vi "_UnitTest.GetDataTypeDescription.vi"() -> ()   [LabVIEW 2014]
panel:
  out "String 12":string
  out "String 16":string
  out "String 11":string
  out "String 15":string
  out "String 14":string
  in  "Digital Data":digitaldata
  out "String 13":string
  in  "Digital Waveform":digitalwaveform(waveform)={"t0"=timestamp(0 s since 1904-01-01), "dt"=1.0, "Y"={"transitions"=[], "data"=[]}}
  out "String 10":string
  in  "Enum":enum16{"a", "b", "c", "d"}(ring)
  out "String 9":string
  in  "Cluster 5":T1
  out "String 8":string
  in  "Cluster 4":T2
  out "String 7":string
  in  "Waveform":waveform(i32)
  out "String 5":string
  in  "Cluster 3":T3
  out "String 4":string
  in  "Cluster 2":T4
  out "String 3":string
  in  "Cluster":cluster{i32, dbl, enum16{""}}
  in  "Array":cluster{i32, dbl, enum16{""}}[](array[cluster])
  in  "Numeric":i32
  out "String 2":string
  out "String":string
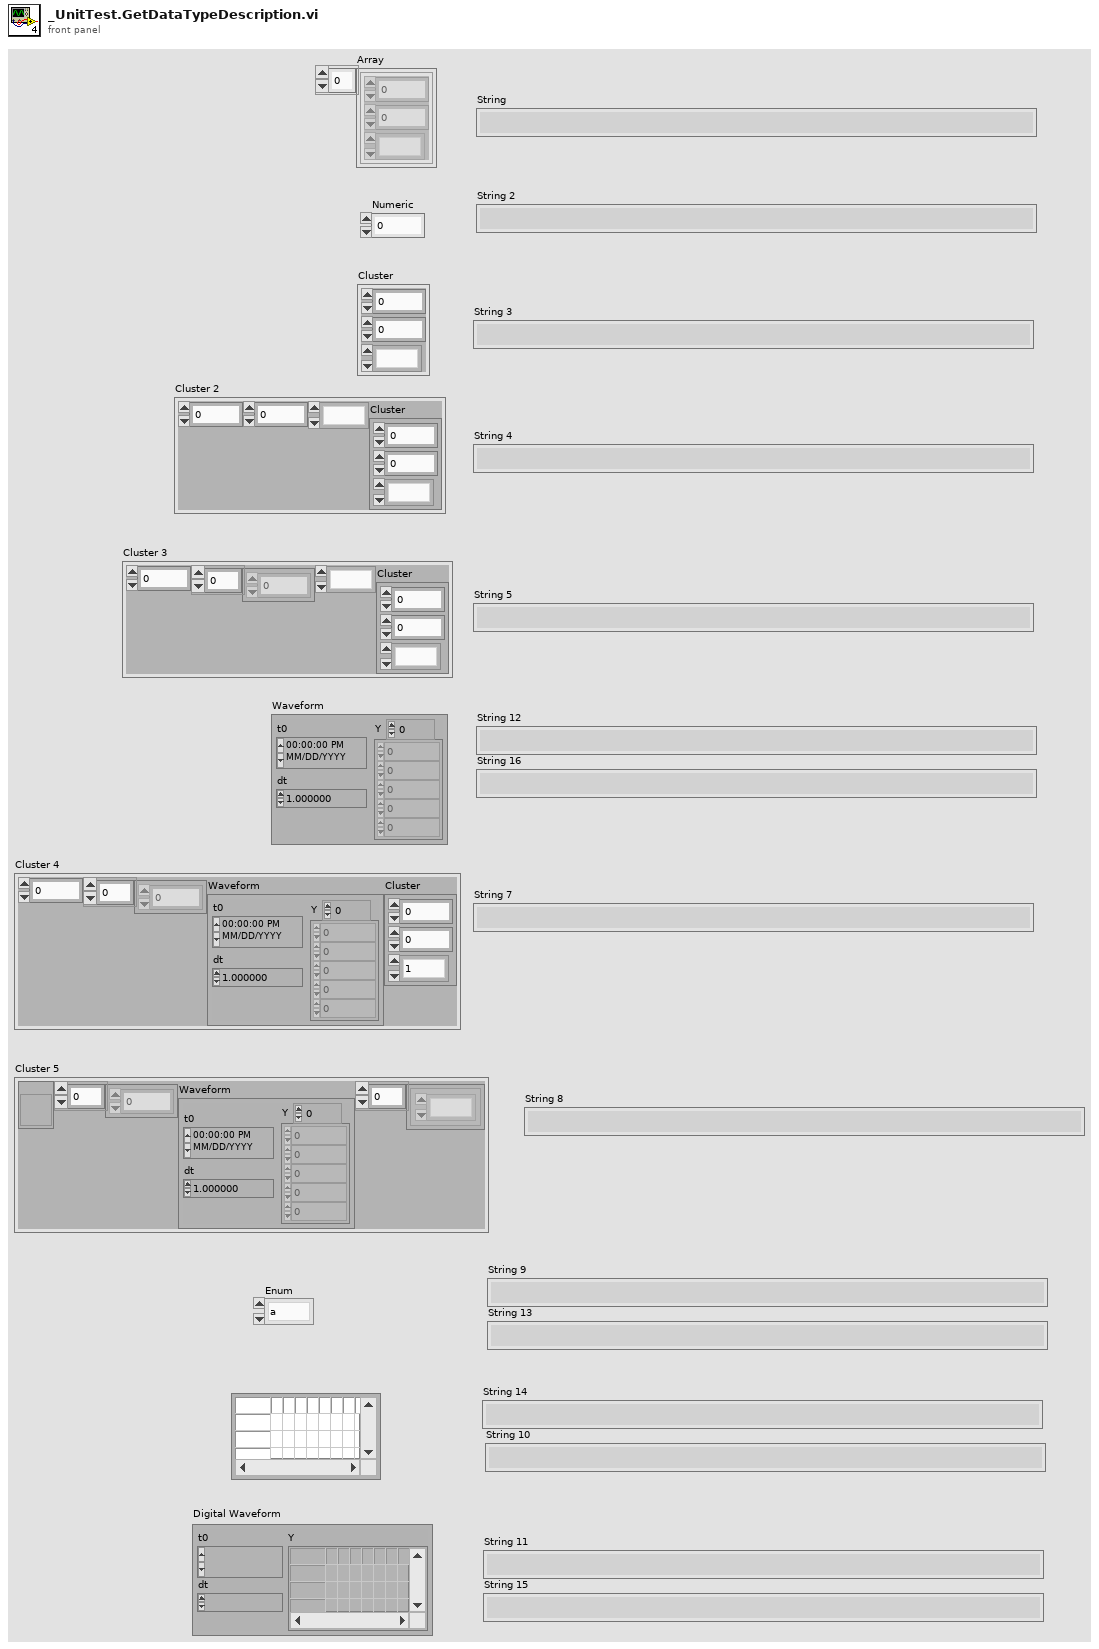
[diagram p1: front panel]
types:
  T1 = cluster{refnum<vi>, dbl[], "Waveform":waveform(dbl), refnum<k1>[]}
  T2 = cluster{i32, dbl[], "Waveform":waveform(dbl), "Cluster":cluster{i32, dbl, enum16{"1", "2", "3"}}}
  T3 = cluster{i32, dbl[], enum16{""}, "Cluster":cluster{i32, dbl, enum16{""}}}
  T4 = cluster{i32, dbl, enum16{""}, "Cluster":cluster{i32, dbl, enum16{""}}}
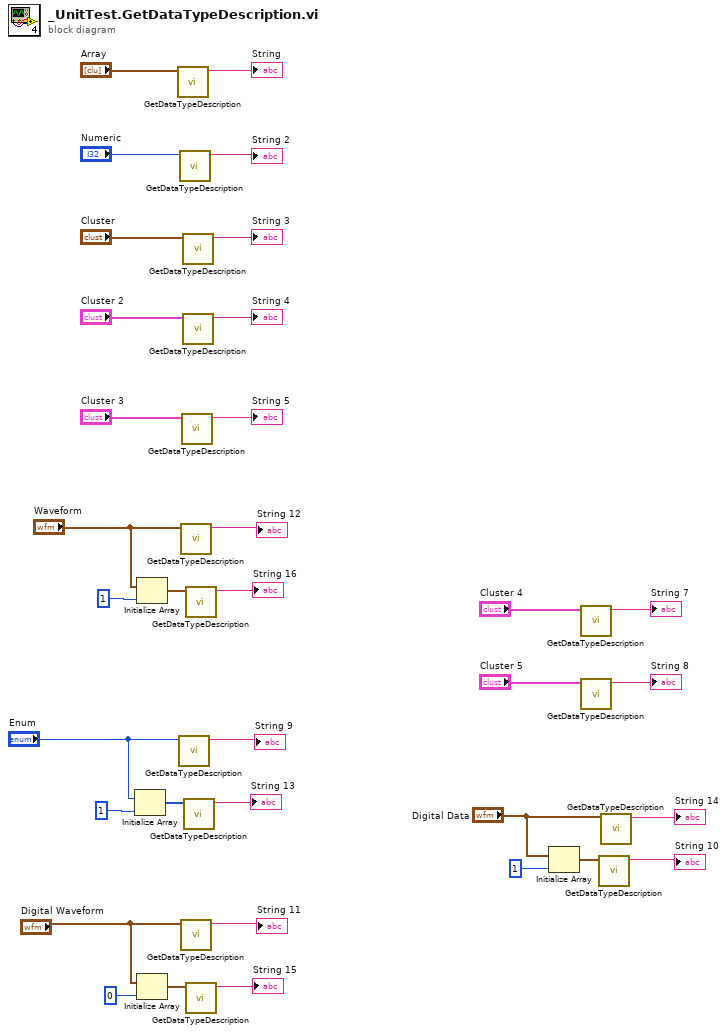
[diagram p0: block diagram]
diagram:
  n1 = Initialize Array("Enum", 1 ("dimension size")) -> (w11:enum16{"a", "b", "c", "d"}[])
  n2 = Initialize Array("Waveform", 1 ("dimension size")) -> (w5:waveform(i32)[])
  n3 = Initialize Array("Digital Waveform", 0 ("dimension size")) -> (w10:digitalwaveform[])
  n4 = call "GetDataTypeDescription.vi"("Variant"="Array") -> ("String"=→"String":string)  [unwired: 9 in, 1 out]
  n5 = call "GetDataTypeDescription.vi"("Variant"="Enum") -> ("String"=→"String 9":string)  [unwired: 9 in, 1 out]
  n6 = call "GetDataTypeDescription.vi"("Variant"="Numeric") -> ("String"=→"String 2":string)  [unwired: 9 in, 1 out]
  n7 = call "GetDataTypeDescription.vi"("Variant"="Waveform") -> ("String"=→"String 12":string)  [unwired: 9 in, 1 out]
  n8 = call "GetDataTypeDescription.vi"("Variant"="Digital Waveform") -> ("String"=→"String 11":string)  [unwired: 9 in, 1 out]
  n9 = call "GetDataTypeDescription.vi"("Variant"="Cluster 3") -> ("String"=→"String 5":string)  [unwired: 9 in, 1 out]
  n10 = call "GetDataTypeDescription.vi"("Variant"="Cluster") -> ("String"=→"String 3":string)  [unwired: 9 in, 1 out]
  n11 = call "GetDataTypeDescription.vi"("Variant"="Cluster 2") -> ("String"=→"String 4":string)  [unwired: 9 in, 1 out]
  n12 = call "GetDataTypeDescription.vi"("Variant"=w11) -> ("String"=→"String 13":string)  [unwired: 9 in, 1 out]
  n13 = call "GetDataTypeDescription.vi"("Variant"=w5) -> ("String"=→"String 16":string)  [unwired: 9 in, 1 out]
  n14 = call "GetDataTypeDescription.vi"("Variant"=w10) -> ("String"=→"String 15":string)  [unwired: 9 in, 1 out]
  n15 = Initialize Array("Digital Data", 1 ("dimension size")) -> (w15:digitaldata[])
  n16 = call "GetDataTypeDescription.vi"("Variant"="Cluster 4") -> ("String"=→"String 7":string)  [unwired: 9 in, 1 out]
  n17 = call "GetDataTypeDescription.vi"("Variant"="Cluster 5") -> ("String"=→"String 8":string)  [unwired: 9 in, 1 out]
  n18 = call "GetDataTypeDescription.vi"("Variant"=w15) -> ("String"=→"String 10":string)  [unwired: 9 in, 1 out]
  n19 = call "GetDataTypeDescription.vi"("Variant"="Digital Data") -> ("String"=→"String 14":string)  [unwired: 9 in, 1 out]
